vi "Process.vi"(8 "error in (no error)":errorcluster, 10 "Pound in":refnum<class "Pound.lvclass">, 11 "Qbus in":refnum<class "Qbus.lvclass">) -> (0 "error out":errorcluster)   [LabVIEW 2017, in "OpState.lvlib"]
doc: "The Trigger process evaluates the expressions that define when a data group enters and exits operating states. After determining the current operating state of the data goup, this process evaluates the file-collection expression for that state to determine whether to collect a file."
uses:
  <vilib>/addons/InsightCM/Devices/Shared/Common/OpState/OpState.lvlib
  <vilib>/addons/Qbus/Qbus.lvclass
  <vilib>/NI/Software Watchdog/Pound/Pound.lvclass
  <vilib>/addons/InsightCM/Devices/Shared/Common/OpState/controls/config.ctl
  <vilib>/addons/InsightCM/MessageBus/MessageLibrary/Tag/controls/TagUpdateStringValuesRoutedMessageBody.ctl
  <vilib>/addons/InsightCM/MessageBus/Base/controls/TagValueString.ctl
  <vilib>/addons/InsightCM/MessageBus/Base/controls/TsTagValueString.ctl
  <vilib>/NI/Software Watchdog/Watchdog/Watchdog.lvclass
  <vilib>/addons/TraceLogger/TraceLogger.lvlib
  <vilib>/addons/InsightCM/Devices/Shared/Common/DataFlow/DataFlow.lvlib
  <vilib>/addons/InsightCM/Devices/Shared/Common/ServerComm/ServerComm.lvlib
  <vilib>/addons/InsightCM/Utilities/GlobalConfiguration/GlobalConfiguration.lvlib
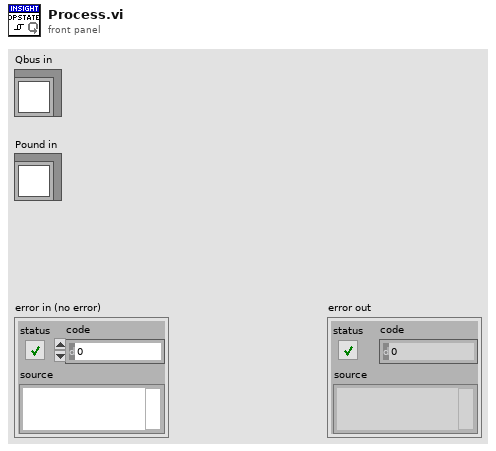
[diagram p1: front panel]
types:
  T1 = typedef "OpState.lvlib/config.ctl" = cluster{"Status":variant, "OpStates":variant, "OpStatesTags":variant, "OpStateTransitionTime":variant}
  T2 = typedef "TagUpdateStringValuesRoutedMessageBody.ctl" = cluster{"TagsValue":T3[]}
  T3 = typedef "TagValueString.ctl" = cluster{"TagId":string, "TsValue":T4}
  T4 = typedef "TsTagValueString.ctl" = cluster{"Value":string, "Timestamp":i64}
  T5 = typedef "DataFlow.lvlib/Data.ctl" = cluster{"DataGroup":string, "Waveforms":T6, "Map":T7, "Type":T8}
  T6 = typedef "wfmSGL_DVR.ctl" = refnum<data-value>
  T7 = typedef "PointValueMap.lvlib/PointMap.ctl" = refnum<data-value>
  T8 = typedef "DataFlow.lvlib/Type.ctl" = enum16{"High Rate", "Low Rate", "Burst Mode"}
  T9 = typedef "ServerComm.lvlib/ConnectionStatus.ctl" = enum16{"Offline", "NotAuthorized", "Online"}
  T10 = typedef "Message.ctl" = cluster{"Header":T11, "Body":u8[]}
  T11 = typedef "MessageHeader.ctl" = cluster{"MessageName":string, "Timestamp":i64, "CorrelationId":string, "ContentType":string, "RoutingKey":string, "Properties":T12[]}
  T12 = typedef "KeyValuePair.ctl" = cluster{"Key":string, "Value":string}
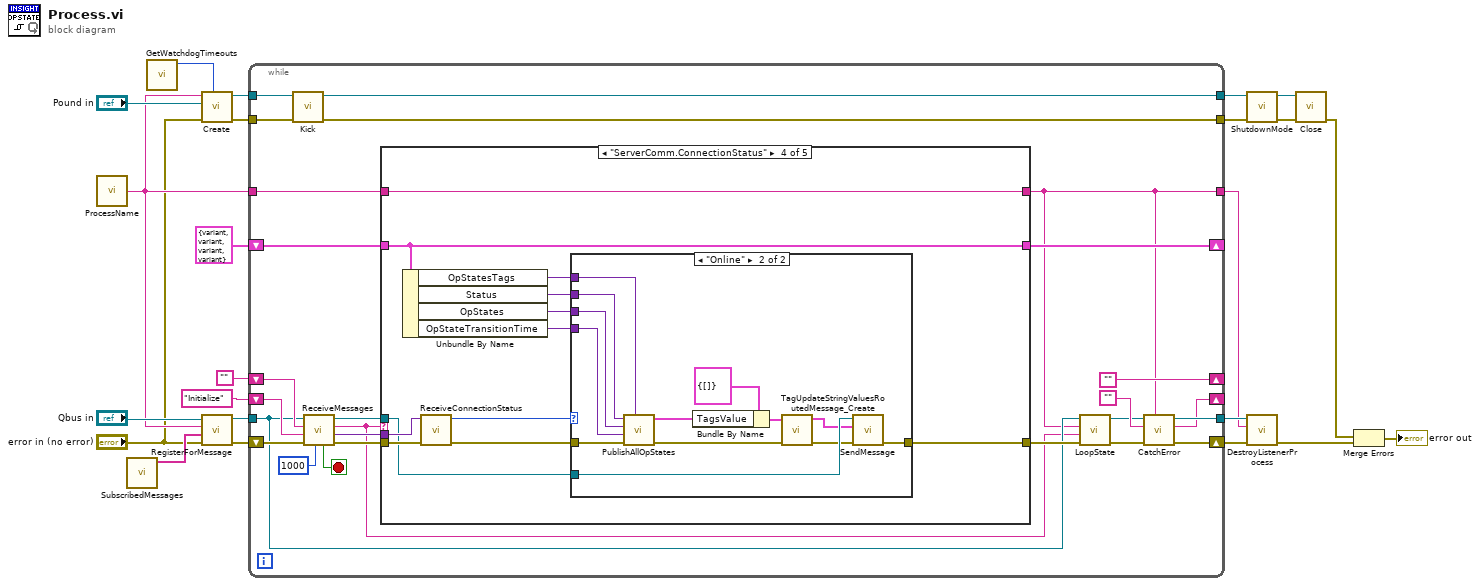
[diagram p0: block diagram]
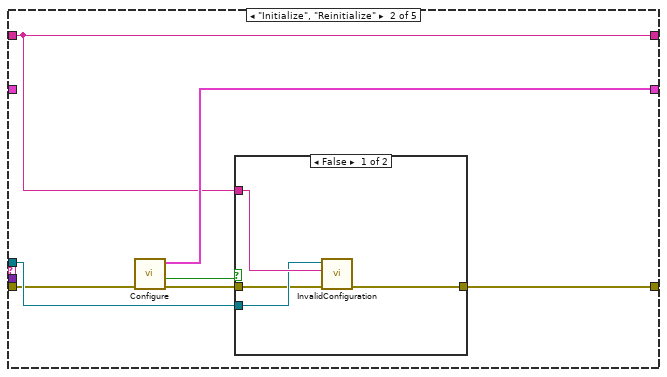
[diagram p3: hidden frame]
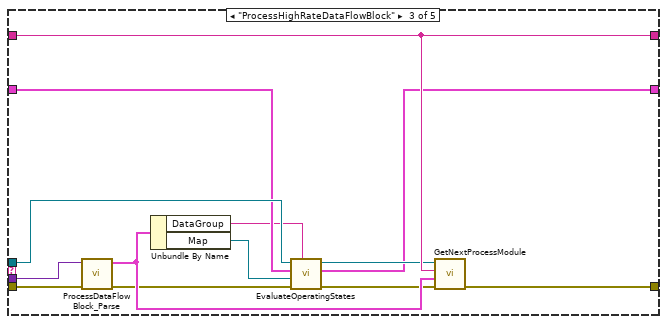
[diagram p5: hidden frame]
diagram:
  n1 = call <vilib>:"ProcessName.vi"() -> ("process name"=w11:string)  [unwired: 5 in]
  n2 = call <vilib>:"SubscribedMessages.vi"() -> ("subscribed messages"=w13:string[])  [unwired: 11 in]
  n3 = call <vilib>:"GetWatchdogTimeouts.vi"() -> ("software timeout"=w1:u32)  [unwired: 10 in, 1 out]
  n4 = call <vilib>:"Create.vi"("Execution Timeout (ms)"=w1, "error in (no error)"="error in (no error)", "Pound"="Pound in", "Name"=w11) -> ("error out"=w10:errorcluster, "Watchdog"=w9:refnum<data-value>)  [unwired: 6 in]
  n5 = call <vilib>:"RegisterForMessage.vi"("error in (no error)"="error in (no error)", "message names"=w13, "process name"=w11, "Qbus in"="Qbus in") -> ("error in (no error)"=w22:errorcluster, "Qbus out"=w21:refnum<class "Qbus.lvclass">)  [unwired: 6 in]
  n6 = while {
    shift-right: [""] -> _
    shift-left: "" -> [w47]
    tunnel: w21 -> [w33]
    tunnel: w11 -> [w35]
    tunnel: [w38] -> w18
    tunnel: [w28] -> w17
    shift-right: [w36] -> _
    shift-left: "Initialize" -> [w42]
    shift-right: [w40] -> _
    shift-left: T1 {"Status"=variant, "OpStates"=variant, "OpStatesTags"=variant, "OpStateTransitionTime"=variant} ("config") -> [w41]
    tunnel: w10 -> [w32]
    tunnel: w9 -> [w31]
    tunnel: [w30] -> w5
    tunnel: [w29] -> w4
    shift-right: [w39] -> w20
    shift-left: w22 -> [w49]
    stop <- w48 stop-if-true
    n7 = call <vilib>:"Kick.vi"("error in (no error)"=w32, "Watchdog"=w31) -> ("error out"=w29:errorcluster, "Watchdog"=w30:refnum<data-value>)  [unwired: 8 in]
    n8 = call <vilib>:"ReceiveMessages.vi"("timeout (1000)"=1000 ("milliseconds to wait"), "error in (no error)"=w49, "priority action"=w42, "default action"=w47, "Qbus in"=w33) -> ("error out"=w46:errorcluster, "message value"=w43:variant, "action"=w27:string, "Qbus out"=w44:refnum<class "Qbus.lvclass">, "exit"=w48:bool)  [unwired: 2 in]
    n9 = case shown="\"ServerComm.ConnectionStatus\"" w27 {
      tunnel: w46 -> [w50 w57 w74 w88 w104]
      tunnel: w44 -> [_ w59 w76 w80 _]
      tunnel: [w50 w58 w77 w81 w104] -> w34
      tunnel: w43 -> [_ _ w73 w87 _]
      tunnel: w41 -> [w52 _ w75 w85 w106]
      tunnel: [w52 w55 w66 w85 w106] -> w40
      tunnel: [w51 w54 w68 w89 w105] -> w28
      tunnel: w35 -> [w51 w54 w68 w89 w105]
      frame "", Default {
      }
      frame "Initialize", "Reinitialize" {
        n10 = call <vilib>:"Configure.vi"("error in (no error)"=w57) -> ("error out"=w56:errorcluster, "valid config"=w53:bool, "config"=w55:T1)  [unwired: 8 in]
        n11 = case shown="False" w53 {
          tunnel: w59 -> [w61 _]
          tunnel: [w63 w64] -> w58
          tunnel: w56 -> [w60 w64]
          tunnel: w54 -> [w62 _]
          frame False {
            n12 = call <vilib>:"InvalidConfiguration.vi"("error in (no error)"=w60, "description"=w62, "Qbus in"=w61) -> ("error out"=w63:errorcluster)  [unwired: 7 in, 1 out]
          }
          frame True {
          }
        }
      }
      frame "ProcessHighRateDataFlowBlock" {
        n13 = call <vilib>:"ProcessDataFlowBlock_Parse.vi"("error in (no error)"=w74, "body"=w73) -> ("error out"=w71:errorcluster, "data"=w72:T5)  [unwired: 8 in]
        n14 = Unbundle By Name(w72) -> ("DataGroup"=w69:string, "Map"=w70:T7)
        n15 = call <vilib>:"EvaluateOperatingStates.vi"("data group"=w69, "error in (no error)"=w71, "map"=w70, "config in"=w75, "Qbus in"=w76) -> ("error out"=w65:errorcluster, "config out"=w66:T1, "Qbus out"=w67:refnum<class "Qbus.lvclass">)  [unwired: 4 in]
        n16 = call <vilib>:"GetNextProcessModule.vi"("error in (no error)"=w65, "data"=w72, "source"=w68, "Qbus in"=w67) -> ("error out"=w77:errorcluster)  [unwired: 6 in, 1 out]
      }
      frame "ServerComm.ConnectionStatus" {
        n17 = Unbundle By Name(w85) -> ("OpStatesTags"=w79:variant, "Status"=w84:variant, "OpStates"=w83:variant, "OpStateTransitionTime"=w82:variant)
        n18 = call <vilib>:"ReceiveConnectionStatus.vi"("error in (no error)"=w88, "body"=w87) -> ("error out"=w86:errorcluster, "status"=w78:T9)  [unwired: 6 in, 2 out]
        n19 = case shown="\"Online\"" w78 {
          tunnel: w86 -> [w90 w103]
          tunnel: w84 -> [_ w102]
          tunnel: w83 -> [_ w101]
          tunnel: w82 -> [_ w100]
          tunnel: [w90 w99] -> w81
          tunnel: w80 -> [_ w98]
          tunnel: w79 -> [_ w97]
          frame "Offline", Default {
          }
          frame "Online" {
            n20 = call <vilib>:"PublishAllOpStates.vi"("OpState tags"=w97, "error in (no error)"=w103, "operating states transition time"=w100, "operating states"=w101, "status"=w102) -> ("error out"=w95:errorcluster, "tag value"=w91:T3[])  [unwired: 5 in]
            n21 = Bundle By Name(cluster=T2 {"TagsValue"=[]} ("TagUpdateStringValuesRoutedMessage"), "TagsValue"=w91) -> (w92:T2)
            n22 = call <vilib>:"TagUpdateStringValuesRoutedMessage_Create.vi"("error in (no error)"=w95, "TagUpdateStringValuesRoutedMessage"=w92) -> ("error out"=w94:errorcluster, "Message"=w93:T10)  [unwired: 8 in]
            n23 = call <vilib>:"SendMessage.vi"("error in (no error)"=w94, "message"=w93, "Qbus in"=w98) -> ("error out"=w99:errorcluster)  [unwired: 7 in, 1 out]
          }
        }
      }
      frame "Exit" {
      }
    }
    n24 = call <vilib>:"LoopState.vi"("error in (no error)"=w34, "loop action"=w27, "process name"=w28, "Qbus in"=w33) -> ("error out"=w25:errorcluster, "Qbus out"=w24:refnum<class "Qbus.lvclass">)  [unwired: 6 in]
    n25 = call <vilib>:"CatchError.vi"("source"=w28, "error in (no error)"=w25, "next action in"="", "Qbus in"=w24) -> ("error out"=w39:errorcluster, "next action out"=w36:string, "Qbus out"=w38:refnum<class "Qbus.lvclass">)  [unwired: 5 in]
  }
  n26 = call <vilib>:"ShutdownMode.vi"("error in (no error)"=w4, "Watchdog"=w5) -> ("error out"=w7:errorcluster, "Watchdog"=w6:refnum<data-value>)  [unwired: 8 in]
  n27 = call <vilib>:"DestroyListenerProcess.vi"("error in (no error)"=w20, "process name"=w17, "Qbus in"=w18) -> ("error in (no error)"=w19:errorcluster)  [unwired: 7 in, 1 out]
  n28 = call <vilib>:"Close.vi"("error in (no error)"=w7, "Watchdog"=w6) -> ("error out"=w2:errorcluster)  [unwired: 9 in]
  n29 = Merge Errors(w2, w19) -> (→"error out":errorcluster)
